vi "labview 4 tania.vi"() -> ()   [LabVIEW 2011]
panel:
  out "Suma 150":dbl
  out "Contador":dbl
  out "Velocidad Promedio":dbl
  out "Velocidad":dbl(knob) scale=0.0..220.0
  # "Generar 10 prueba de velocidad \nluego sumar las velocidades\nmayores a 150 y obtener su promedio."
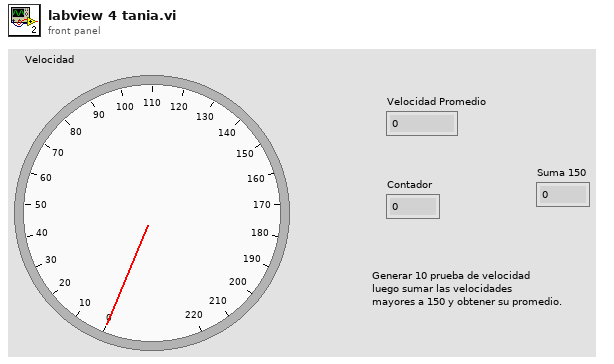
[diagram p1: front panel]
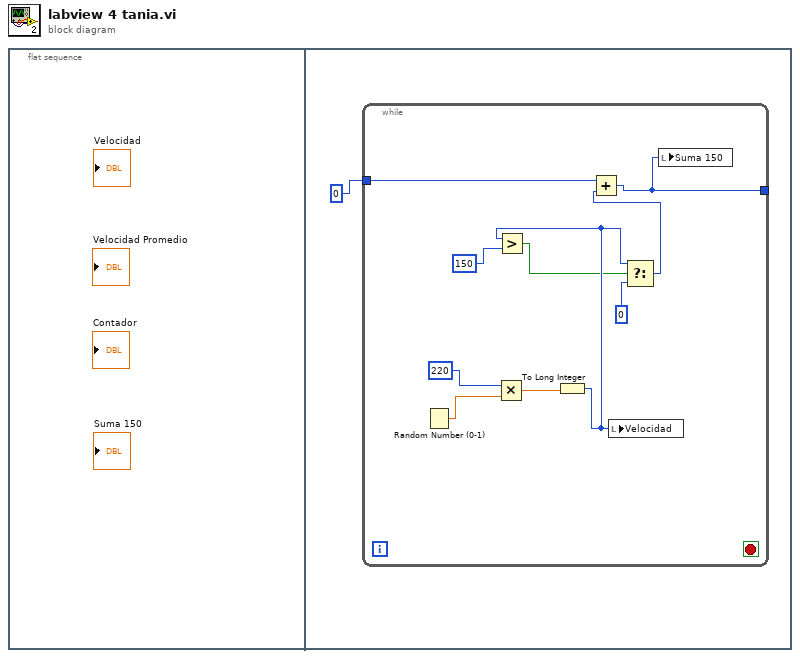
[diagram p0: block diagram]
diagram:
  n1 = flat-sequence {
    frame #0 {
    }
    frame #1 {
      n2 = while {
        tunnel: 0 -> [w11]
        tunnel: [w2] -> _
        stop <- _ stop-if-true
        n3 = Random Number (0-1)() -> (number: 0 to 1=w9:dbl)
        n4 = Multiply(x=220, y=w9) -> (x*y=w8:dbl)
        n5 = To Long Integer(number=w8) -> (32bit integer=w5:i32)
        n6 = Greater?(x=w5, y=150) -> (0:w4:bool)
        n7 = local write "Velocidad"(w5) -> ()
        n8 = Select(t=w5, s=w4, f=0) -> (s? t:f=w3:i32)
        n9 = Add(x=w11, y=w3) -> (x+y=w2:i32)
        n10 = local write "Suma 150"(w2) -> ()
      }
    }
  }
